vi "extract address and function code.vi"(11 "Cmd to Send":string) -> (1 "Function Code":string, 3 "SendAddress":string)   [LabVIEW 2014, in "HPCNC.lvlib"]
uses:
  HPCNC.lvlib
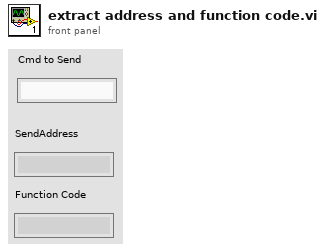
[diagram p1: front panel]
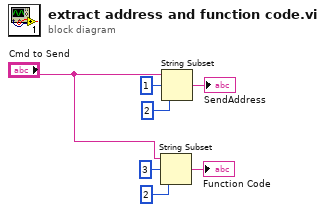
[diagram p0: block diagram]
diagram:
  n1 = String Subset(string="Cmd to Send", offset (0)=3, length (rest)=2 ("length (rest)")) -> (substring=→"Function Code":string)
  n2 = String Subset(string="Cmd to Send", offset (0)=1, length (rest)=2 ("length (rest)")) -> (substring=→"SendAddress":string)
